vi "STD_MeasureInfoToModType.vi"(11 "MeasureInfo":T1 {"MeasStopInfo"."flags" format="x%x"; "MeasureInfo_PartB"."mod_type2" format="%016x"; "MeasureInfo_PartB"."mod_type1" format="%.0x"}) -> (3 "mod_type":string)   [LabVIEW 2017]
uses:
  SPC_Wrappers/SPC_Controls/MeasureInfo.ctl
  SPC_Wrappers/SPC_Controls/MeasureInfo_PartB.ctl
  SPC_Wrappers/SPC_Controls/MeasStopInfo.ctl
  SPC_Wrappers/SPC_Controls/MeasFCSInfo.ctl
  SPC_Wrappers/SPC_Controls/MeasureInfo_PartE.ctl
  SPC_Wrappers/SPC_Controls/MeasHISTInfo.ctl
  SPC_Wrappers/SPC_Controls/HISTInfoExt.ctl
  SPC_Wrappers/SPC_Controls/MeasureInfo_PartI.ctl
  SPC_Wrappers/SPC_Controls/MeasureInfo_PartK.ctl
  SPC_Wrappers/SPC_Controls/MeasureInfo_PartM.ctl
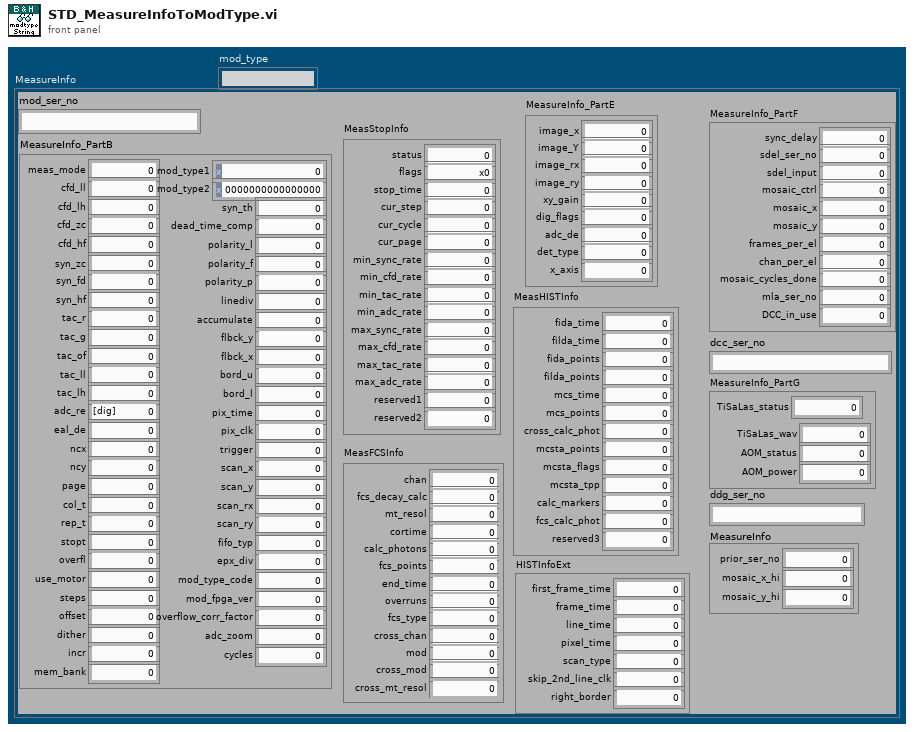
[diagram p1: front panel]
types:
  T1 = typedef "MeasureInfo.ctl" = cluster{"mod_ser_no":string, "MeasureInfo_PartB":T2, "MeasStopInfo":T3, "MeasFCSInfo":T4, "MeasureInfo_PartE":T5, "MeasHISTInfo":T6, "HISTInfoExt":T7, "MeasureInfo_PartF":T8, "dcc_ser_no":string, "MeasureInfo_PartG":T9, "ddg_ser_no":string, "MeasureInfo":T10}
  T2 = typedef "MeasureInfo_PartB.ctl" = cluster{"meas_mode":i16, "cfd_ll":sgl, "cfd_lh":sgl, "cfd_zc":sgl, "cfd_hf":sgl, "syn_zc":sgl, "syn_fd":i16, "syn_hf":sgl, "tac_r":sgl, "tac_g":i16, "tac_of":sgl, "tac_ll":sgl, "tac_lh":sgl, "adc_re":i16, "eal_de":i16, "ncx":i16, "ncy":i16, "page":u16, "col_t":sgl, "rep_t":sgl, "stopt":i16, "overfl":i8, "use_motor":i16, "steps":u16, "offset":sgl, "dither":i16, "incr":i16, "mem_bank":i16, "mod_type1":u64, "mod_type2":u64, "syn_th":sgl, "dead_time_comp":i16, "polarity_l":i16, "polarity_f":i16, "polarity_p":i16, "linediv":i16, "accumulate":i16, "flbck_y":i32, "flbck_x":i32, "bord_u":i32, "bord_l":i32, "pix_time":sgl, "pix_clk":i16, "trigger":i16, "scan_x":i32, "scan_y":i32, "scan_rx":i32, "scan_ry":i32, "fifo_typ":i16, "epx_div":i32, "mod_type_code":u16, "mod_fpga_ver":u16, "overflow_corr_factor":sgl, "adc_zoom":i32, "cycles":i32}
  T3 = typedef "MeasStopInfo.ctl" = cluster{"status":u16, "flags":u16, "stop_time":sgl, "cur_step":i32, "cur_cycle":i32, "cur_page":i32, "min_sync_rate":sgl, "min_cfd_rate":sgl, "min_tac_rate":sgl, "min_adc_rate":sgl, "max_sync_rate":sgl, "max_cfd_rate":sgl, "max_tac_rate":sgl, "max_adc_rate":sgl, "reserved1":i32, "reserved2":sgl}
  T4 = typedef "MeasFCSInfo.ctl" = cluster{"chan":u16, "fcs_decay_calc":u16, "mt_resol":u32, "cortime":sgl, "calc_photons":u32, "fcs_points":i32, "end_time":sgl, "overruns":u16, "fcs_type":u16, "cross_chan":u16, "mod":u16, "cross_mod":u16, "cross_mt_resol":u32}
  T5 = typedef "MeasureInfo_PartE.ctl" = cluster{"image_x":i32, "image_Y":i32, "image_rx":i32, "image_ry":i32, "xy_gain":i16, "dig_flags":i16, "adc_de":i16, "det_type":i16, "x_axis":i16}
  T6 = typedef "MeasHISTInfo.ctl" = cluster{"fida_time":sgl, "filda_time":sgl, "fida_points":i32, "filda_points":i32, "mcs_time":sgl, "mcs_points":i32, "cross_calc_phot":u32, "mcsta_points":u16, "mcsta_flags":u16, "mcsta_tpp":u32, "calc_markers":u32, "fcs_calc_phot":u32, "reserved3":u32}
  T7 = typedef "HISTInfoExt.ctl" = cluster{"first_frame_time":sgl, "frame_time":sgl, "line_time":sgl, "pixel_time":sgl, "scan_type":i16, "skip_2nd_line_clk":i16, "right_border":u32}
  T8 = typedef "MeasureInfo_PartI.ctl" = cluster{"sync_delay":sgl, "sdel_ser_no":u16, "sdel_input":i8, "mosaic_ctrl":i8, "mosaic_x":u8, "mosaic_y":u8, "frames_per_el":i16, "chan_per_el":i16, "mosaic_cycles_done":i32, "mla_ser_no":u16, "DCC_in_use":u8}
  T9 = typedef "MeasureInfo_PartK.ctl" = cluster{"TiSaLas_status":u16, "TiSaLas_wav":u16, "AOM_status":u8, "AOM_power":u8}
  T10 = typedef "MeasureInfo_PartM.ctl" = cluster{"prior_ser_no":i32, "mosaic_x_hi":u8, "mosaic_y_hi":u8}
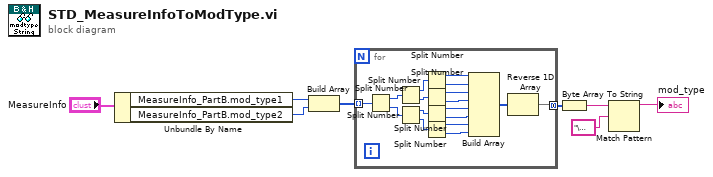
[diagram p0: block diagram]
diagram:
  n1 = Unbundle By Name("MeasureInfo") -> ("MeasureInfo_PartB.mod_type1"=w7:u64, "MeasureInfo_PartB.mod_type2"=w5:u64)
  n2 = Build Array(w7, w5) -> (w6:u64[])
  n3 = for {
    tunnel: [w9] -> w4 mode=concatenating
    tunnel: w6 -> [w10] mode=indexing
    n4 = Split Number(x=w10) -> (hi(x)=w25:u32, lo(x)=w24:u32)
    n5 = Split Number(x=w25) -> (hi(x)=w23:u16, lo(x)=w22:u16)
    n6 = Split Number(x=w24) -> (hi(x)=w21:u16, lo(x)=w20:u16)
    n7 = Split Number(x=w23) -> (hi(x)=w19:u8, lo(x)=w18:u8)
    n8 = Split Number(x=w22) -> (hi(x)=w17:u8, lo(x)=w16:u8)
    n9 = Split Number(x=w21) -> (hi(x)=w15:u8, lo(x)=w14:u8)
    n10 = Split Number(x=w20) -> (hi(x)=w13:u8, lo(x)=w12:u8)
    n11 = Build Array(w19, w18, w17, w16, w15, w14, w13, w12) -> (w11:u8[])
    n12 = Reverse 1D Array(array=w11) -> (reversed array=w9:u8[])
  }
  n13 = Byte Array To String(unsigned byte array=w4) -> (string=w3:string)
  n14 = Match Pattern(string=w3, regular expression="\u0000") -> (before substring=→"mod_type":string)  [unwired: 1 in, 3 out]
